vi "XML Parse.vi"(8 "error in (no error)":errorcluster, 9 "Name String":string, 10 "Type String":string, 11 "Path":path) -> (0 "error out":errorcluster, 2 "String Out":string)   [LabVIEW 2009]
uses:
  <vilib>/xml/Load XML File.vi
  <vilib>/xml/NI_XML.lvlib
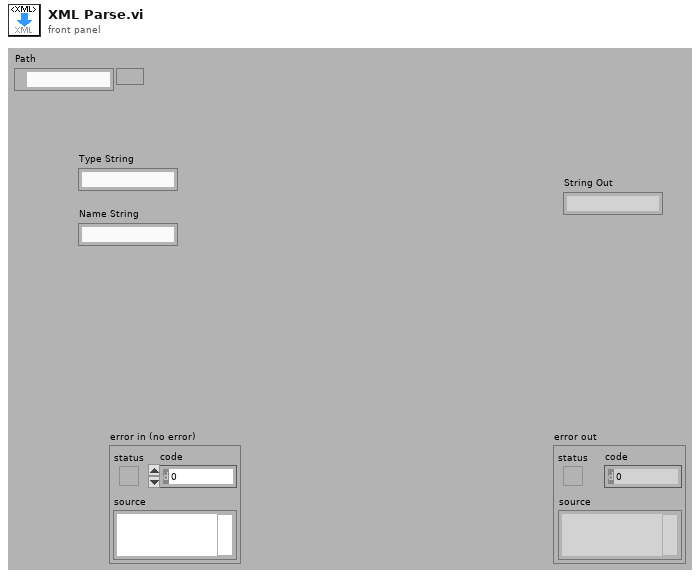
[diagram p1: front panel]
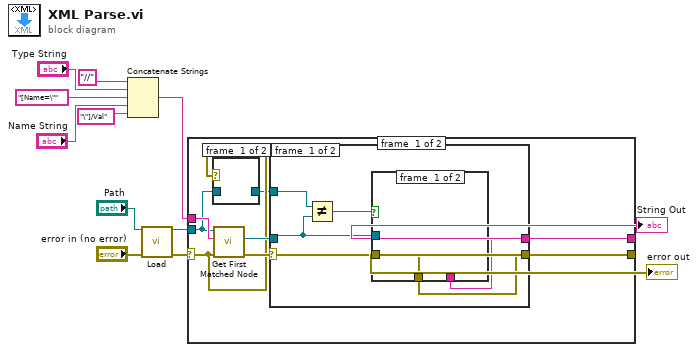
[diagram p0: block diagram]
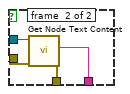
[diagram p3: hidden frame]
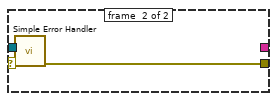
[diagram p4: hidden frame]
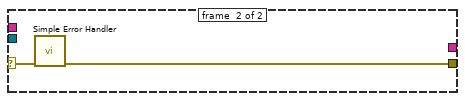
[diagram p5: hidden frame]
diagram:
  n1 = Concatenate Strings("//", "Type String", "[Name=\"", "Name String", "\"]/Val") -> (w6:string)
  n2 = call-poly <vilib>:"Load.vi"("path to XML document"="Path", "error in (no error)"="error in (no error)") -> ("DOM document out"=w7:refnum<k20>, "error out"=w3:errorcluster)  [unwired: 11 in, 1 out]
  n3 = case shown="No Error" w3 {
    selector: w3 -> [w14 w36]
    tunnel: w7 -> [w15 _]
    tunnel: w6 -> [w19 _]
    tunnel: [w17 _] -> w1
    tunnel: [w16 w35] -> w2
    frame #0 {
      n4 = case shown="No Error" w14 {
        tunnel: w15 -> [_ w21]
        tunnel: [_ w21] -> w13
        frame #0 {
        }
        frame #1 {
        }
      }
      n5 = call <vilib>:"Get First Matched Node.vi"("error in (no error)"=w14, "XPath expression"=w19, "node in"=w15) -> ("error out"=w18:errorcluster, "node result"=w20:refnum<k20>)  [unwired: 6 in, 1 out]
      n6 = case shown="No Error" w18 {
        selector: w18 -> [w27 w34]
        tunnel: w20 -> [w23 _]
        tunnel: [w26 _] -> w17
        tunnel: [w25 w33] -> w16
        tunnel: w13 -> [w24 _]
        frame #0 {
          n7 = Not Equal?(x=w24, y=w23) -> (x != y?=w22:bool)
          n8 = case shown="False" w22 {
            tunnel: w23 -> [_ w32]
            tunnel: w27 -> [w28 w31]
            tunnel: [_ w30] -> w26
            tunnel: [w28 w29] -> w25
            frame #0 {
            }
            frame #1 {
              n9 = call <vilib>:"Get Node Text Content.vi"("error in (no error)"=w31, "node in"=w32) -> ("error out"=w29:errorcluster, "node text"=w30:string)  [unwired: 7 in, 1 out]
            }
          }
        }
        frame #1 {
          n10 = call <vilib>:"Simple Error Handler.vi"("error in (no error)"=w34) -> ("error out"=w33:errorcluster)  [unwired: 4 in, 4 out]
        }
      }
    }
    frame #1 {
      n11 = call <vilib>:"Simple Error Handler.vi"("error in (no error)"=w36) -> ("error out"=w35:errorcluster)  [unwired: 4 in, 4 out]
    }
  }
  "error out" <- w2
  "String Out" <- w1
